vi "oa_FIR Preprocess Filter Kaiser Parameter.vi"(6 "fs [Hz]":dbl, 8 "error in (no error)":errorcluster, 9 "A stop":dbl, 11 "delta f [Hz]":dbl) -> (0 "error out":errorcluster, 2 "beta":dbl, 3 "estimated order":i32)   [LabVIEW 2017, in "SoundVib_RefDataProcess.lvlib"]
uses:
  <vilib>/addons/Sound and Vibration/Order Analysis/Referece Data Processing/SoundVib_RefDataProcess.lvlib
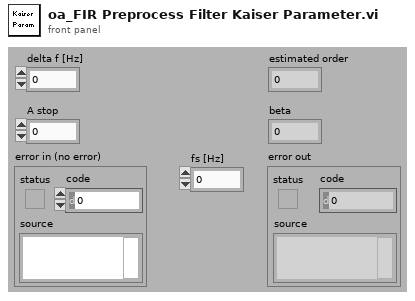
[diagram p1: front panel]
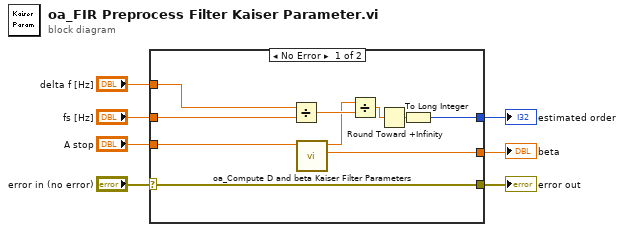
[diagram p0: block diagram]
diagram:
  n1 = case shown="No Error" "error in (no error)" {
    selector: "error in (no error)" -> [w14 w18]
    tunnel: "delta f [Hz]" -> [w17 _]
    tunnel: "fs [Hz]" -> [w16 _]
    tunnel: "A stop" -> [w8 _]
    tunnel: [w11 _] -> w4
    tunnel: [w15 _] -> w3
    tunnel: [w14 w18] -> w1
    frame No Error {
      n2 = Divide(x=w17, y=w16) -> (x/y=w10:dbl)
      n3 = call <vilib>:"oa_Compute D and beta Kaiser Filter Parameters.vi"("A stop"=w8) -> ("beta"=w15:dbl, "D"=w9:dbl)  [unwired: 9 in]
      n4 = Divide(x=w9, y=w10) -> (x/y=w13:dbl)
      n5 = Round Toward +Infinity(x=w13) -> (ceil(x): smallest int >= x=w12:dbl)
      n6 = To Long Integer(number=w12) -> (32bit integer=w11:i32)
    }
    frame Error {
    }
  }
  "estimated order" <- w4
  "beta" <- w3
  "error out" <- w1
